vi "Data Parser.vi"(10 "String":string) -> (0 "Stable?":bool, 1 "NET":bool, 2 "Units":string, 3 "Value":dbl format="%.2g")   [LabVIEW 2015, in "Ohaus AV Series.lvlib"]
doc: "This VI takes the output of the instrument and converts it to a numeric value, and units. It also tells if the value was stable when taken and if a tare is present (NET) The data must only be one line in the form"
uses:
  Ohaus AV Series.lvlib
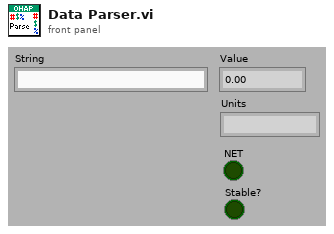
[diagram p1: front panel]
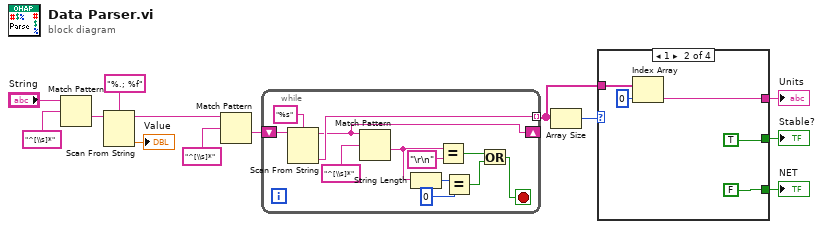
[diagram p0: block diagram]
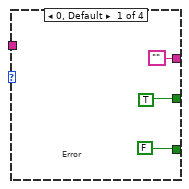
[diagram p2: hidden frame]
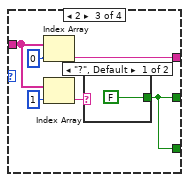
[diagram p3: hidden frame]
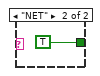
[diagram p4: hidden frame]
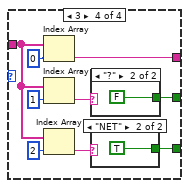
[diagram p5: hidden frame]
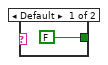
[diagram p6: hidden frame]
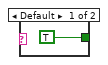
[diagram p7: hidden frame]
diagram:
  n1 = Match Pattern(string="String", regular expression="^[\\s]*") -> (after substring=w10:string)  [unwired: 1 in, 3 out]
  n2 = Scan From String(format string="%.; %f", input string=w10) -> (remaining string=w7:string, output 1=→"Value":dbl)  [unwired: 3 in, 2 out]
  n3 = Match Pattern(string=w7, regular expression="^[\\s]*") -> (after substring=w6:string)  [unwired: 1 in, 3 out]
  n4 = while {
    tunnel: [w15] -> w4 mode=indexing
    shift-right: [w14] -> _
    shift-left: w6 -> [w24]
    stop <- w16 stop-if-true
    n5 = Scan From String(format string="%s", input string=w24) -> (remaining string=w14:string, output 1=w15:string)  [unwired: 3 in, 2 out]
    n6 = Match Pattern(string=w14, regular expression="^[\\s]*") -> (after substring=w20:string)  [unwired: 1 in, 3 out]
    n7 = String Length(string=w20) -> (length=w19:i32)
    n8 = Equal?(x=w20, y="\r\n") -> (x = y?=w21:bool)
    n9 = Equal?(x=w19, y=0) -> (x = y?=w17:bool)
    n10 = Or(x=w21, y=w17) -> (x .or. y?=w16:bool)
  }
  n11 = Array Size(array=w4) -> (size(s)=w5:i32)
  n12 = case shown="1" w5 {
    tunnel: w4 -> [_ w33 w39 w47]
    tunnel: ["" w31 w36 w46] -> w3
    tunnel: [TRUE TRUE w34 w44] -> w1
    tunnel: [FALSE FALSE w34 w42] -> w2
    frame 0, Default {
      # "Error"
    }
    frame 1 {
      n13 = Index Array(array=w33, index=0) -> (element=w31:string)
    }
    frame 2 {
      n14 = Index Array(array=w39, index=0) -> (element=w36:string)
      n15 = Index Array(array=w39, index=1) -> (element=w35:string)
      n16 = case shown="\"?\", Default" w35 {
        tunnel: [FALSE TRUE] -> w34
        frame "?", Default {
        }
        frame "NET" {
        }
      }
    }
    frame 3 {
      n17 = Index Array(array=w47, index=0) -> (element=w46:string)
      n18 = Index Array(array=w47, index=1) -> (element=w45:string)
      n19 = Index Array(array=w47, index=2) -> (element=w43:string)
      n20 = case shown="\"?\"" w45 {
        tunnel: [TRUE FALSE] -> w44
        frame Default {
        }
        frame "?" {
        }
      }
      n21 = case shown="\"NET\"" w43 {
        tunnel: [FALSE TRUE] -> w42
        frame Default {
        }
        frame "NET" {
        }
      }
    }
  }
  "Units" <- w3
  "NET" <- w2
  "Stable?" <- w1
